vi "Analog Output Write.vi"(8 "error in (no error)":errorcluster, 10 "Analog Output Write":dbl[](array[numeric]) format="%0.2f", 11 "AO in":refnum<class "AO.lvclass">) -> (0 "error out":errorcluster, 3 "AO out":refnum<class "AO.lvclass">)   [LabVIEW 2023, in "HardwareAbstractionLayer_LVOOP.lvlib" / "AO.lvclass"]
uses:
  AO.lvclass
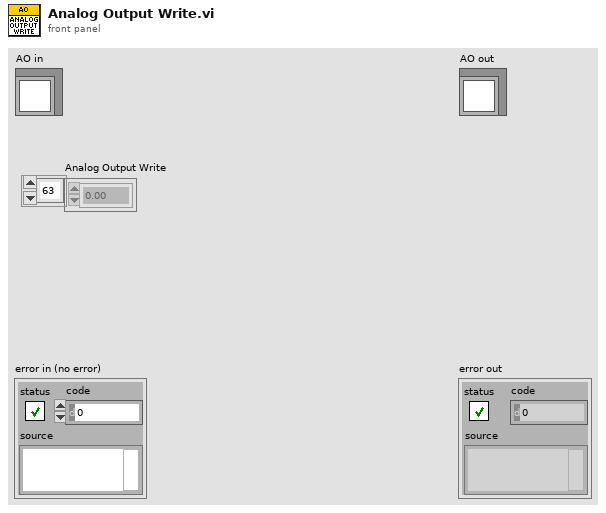
[diagram p1: front panel]
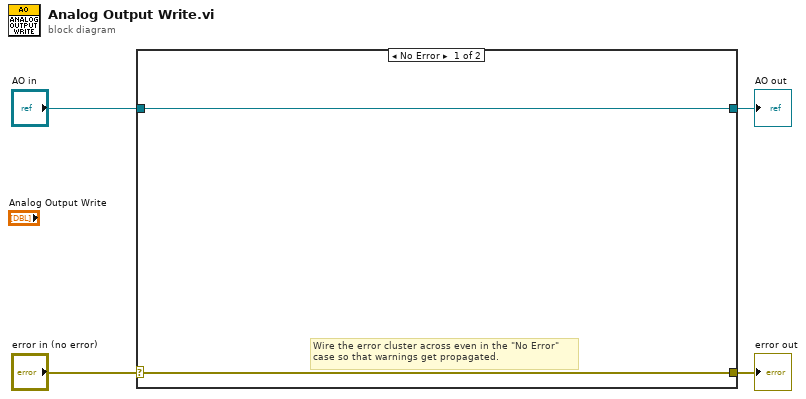
[diagram p0: block diagram]
diagram:
  n1 = case shown="No Error" "error in (no error)" {
    selector: "error in (no error)" -> [w5 w8]
    tunnel: [w5 w8] -> w3
    tunnel: [w6 w7] -> w1
    tunnel: "AO in" -> [w6 w7]
    frame No Error {
      # "Wire the error cluster across even in the \"No Error\"\ncase so that warnings get propagated."
    }
    frame Error {
    }
  }
  "error out" <- w3
  "AO out" <- w1
